vi "Is DaisyChain open.vi"(0 "System no.":i32=1 min=1 step=1, 5 "error in":errorcluster) -> (14 "PortID":i32, 15 "DC open?":bool, 19 "error out":errorcluster)   [LabVIEW 2020]
doc: "This VI checks if a DaisyChain connection is already open for the communication port defined for the given System no. It does also return the Port ID of the DaisyChain connection if any exists.\n\nE-709: Only supported if E-709 is used inside C-867K012/K013."
uses:
  ProgramData/PI/LabVIEW/Low Level/Communication.llb/Global DaisyChain.vi
  ProgramData/PI/LabVIEW/Low Level/Communication.llb/Global1.vi
panel:
  # "This vi checks if a DaisyChain connection is already open \nfor the selected interface."
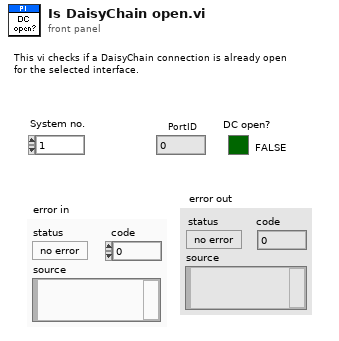
[diagram p1: front panel]
types:
  T1 = typedef "Available DLLs.ctl" = u16
  T2 = typedef "Available DLL interfaces.ctl" = u16
  T3 = cluster{"DLL for Device":T1, "DLL Interface":T2, "Parameter":string}[]
  T4 = typedef "Available interfaces.ctl" = u16
  T5 = cluster{"RS232 Portnumber":i32, "Timeout":i32, "RS232 Baud rate":u32, "Interface":T4, "GPIB Bus":i32, "GPIB Address":i32, "GPIB Mode":i32}[]
  T6 = cluster{"No. of devices":i32, "Port ID":i32, "Devices":string[], "Description":string}[]
  T7 = cluster{"RS232 Portnumber":i32, "Timeout":i32, "RS232 Baud rate":u32, "Interface":T4, "GPIB Bus":i32, "GPIB Address":i32, "GPIB Mode":i32}
  T8 = cluster{"DLL for Device":T1, "DLL Interface":T2, "Parameter":string}
  T9 = cluster{"No. of devices":i32, "Port ID":i32, "Devices":string[], "Description":string}
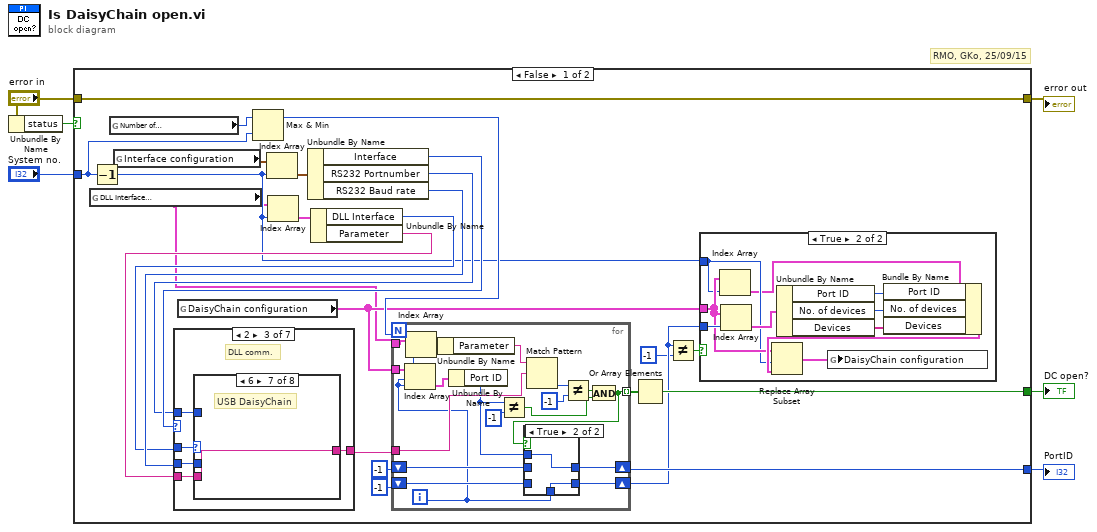
[diagram p0: block diagram]
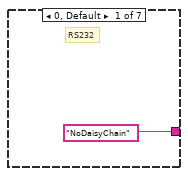
[diagram p3: hidden frame]
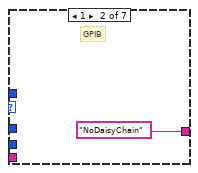
[diagram p4: hidden frame]
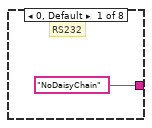
[diagram p5: hidden frame]
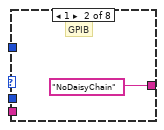
[diagram p6: hidden frame]
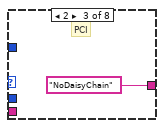
[diagram p7: hidden frame]
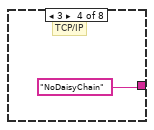
[diagram p8: hidden frame]
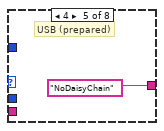
[diagram p9: hidden frame]
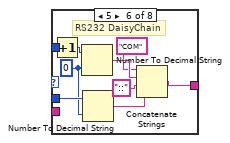
[diagram p10: hidden frame]
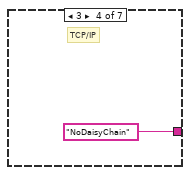
[diagram p12: hidden frame]
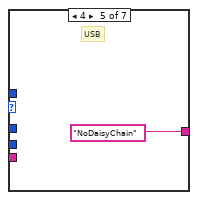
[diagram p13: hidden frame]
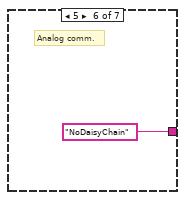
[diagram p14: hidden frame]
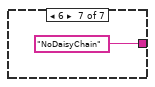
[diagram p15: hidden frame]
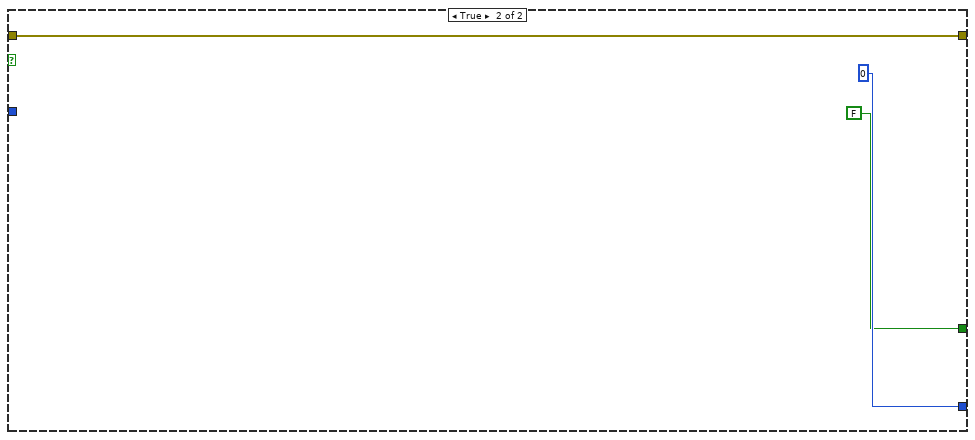
[diagram p17: hidden frame]
diagram:
  # "RMO, GKo, 25/09/15"
  n1 = Unbundle By Name("error in") -> ("status"=w5:bool)
  n2 = case shown="False" w5 {
    tunnel: [w22 w92] -> w4
    tunnel: "error in" -> [w22 w92]
    tunnel: [w26 0] -> w3
    tunnel: [w14 FALSE] -> w2
    tunnel: "System no." -> [w17 _]
    frame False {
      n3 = global read "Global1.vi" "DLL Interface\nConfiguration"() -> (w7:T3)
      n4 = Decrement(x=w17) -> (x-1=w8:i32)
      n5 = global read "Global1.vi" "Number of\nsystems"() -> (w18:i32)
      n6 = global read "Global1.vi" "Interface configuration"() -> (w30:T5)
      n7 = global read "Global DaisyChain.vi" "DaisyChain configuration"() -> (w9:T6)
      n8 = Max & Min(x=w18, y=w17) -> (max(x,y)=w16:i32)  [unwired: 1 out]
      n9 = Index Array(array=w30, index=w8) -> (element=w29:T7)
      n10 = Index Array(array=w7, index=w8) -> (element=w21:T8)
      n11 = Unbundle By Name(w29) -> ("Interface"=w25:T4, "RS232 Portnumber"=w24:i32, "RS232 Baud rate"=w23:u32)
      n12 = Unbundle By Name(w21) -> ("DLL Interface"=w20:T2, "Parameter"=w10:string)
      n13 = case shown="2" w25 {
        tunnel: ["NoDaisyChain" "NoDaisyChain" w47 "NoDaisyChain" "NoDaisyChain" "NoDaisyChain" "NoDaisyChain"] -> w19
        tunnel: w24 -> [_ _ w46 _ _ _ _]
        tunnel: w23 -> [_ _ w45 _ _ _ _]
        tunnel: w20 -> [_ _ w44 _ _ _ _]
        tunnel: w10 -> [_ _ w43 _ _ _ _]
        frame 0, Default {
          # "RS232"
        }
        frame 1 {
          # "GPIB"
        }
        frame 2 {
          # "DLL comm."
          n14 = case shown="6" w44 {
            tunnel: ["NoDaisyChain" "NoDaisyChain" "NoDaisyChain" "NoDaisyChain" "NoDaisyChain" w58 w62 w63] -> w47
            tunnel: w46 -> [_ _ _ _ _ w57 _ _]
            tunnel: w45 -> [_ _ _ _ _ w55 _ _]
            tunnel: w43 -> [_ _ _ _ _ _ w62 w63]
            frame 0, Default {
              # "RS232"
            }
            frame 1 {
              # "GPIB"
            }
            frame 2 {
              # "PCI"
            }
            frame 3 {
              # "TCP/IP"
            }
            frame 4 {
              # "USB (prepared)"
            }
            frame 5 {
              w54 = i16 0 ("width (-)")
              # "RS232 DaisyChain"
              n15 = Increment(x=w57) -> (x+1=w56:i32)
              n16 = Number To Decimal String(number=w56, width (-)=w54) -> (decimal integer string=w61:string)
              n17 = Number To Decimal String(number=w55, width (-)=w54) -> (decimal integer string=w59:string)
              n18 = Concatenate Strings("COM" ("string"), w61, "::" ("string"), w59) -> (w58:string)
            }
            frame 6 {
              # "USB DaisyChain"
            }
            frame 7 {
              # "TCPIP DaisyChain"
            }
          }
        }
        frame 3 {
          # "TCP/IP"
        }
        frame 4 {
          (unwired) refnum<visa-resource-name> refnum ("duplicate VISA resource name")
          (unwired) FALSE ("status")
          (unwired) 0 ("error code")
          (unwired) 0
          # "USB"
        }
        frame 5 {
          (unwired) refnum<visa-resource-name> refnum ("duplicate VISA resource name")
          (unwired) FALSE ("status")
          (unwired) 0 ("error code")
          (unwired) 0
          # "Analog comm."
        }
        frame 6 {
        }
      }
      n19 = for {
        N: w16 -> [_]
        tunnel: w9 -> [w73]
        tunnel: [w79] -> w28 mode=indexing
        shift-right: [w83] -> w26
        shift-left: -1 ("Port ID") -> [w82]
        tunnel: w19 -> [w81]
        shift-right: [w74] -> w13
        shift-left: -1 -> [w75]
        tunnel: w7 -> [w71]
        i -> [w72]
        n20 = Index Array(array=w73, index=w72) -> (element=w70:T9)
        n21 = Index Array(array=w71, index=w72) -> (element=w69:T8)
        n22 = Unbundle By Name(w69) -> ("Parameter"=w68:string)
        n23 = Unbundle By Name(w70) -> ("Port ID"=w77:i32)
        n24 = Not Equal?(x=w77, y=-1) -> (x != y?=w76:bool)
        n25 = Match Pattern(string=w68, regular expression=w81) -> (offset past match=w85:i32)  [unwired: 4 out]
        n26 = Not Equal?(x=w85, y=-1) -> (x != y?=w80:bool)
        n27 = And(x=w80, y=w76) -> (x .and. y?=w79:bool)
        n28 = case shown="True" w79 {
          tunnel: [w87 w89] -> w83
          tunnel: w77 -> [_ w89]
          tunnel: w82 -> [w87 _]
          tunnel: w75 -> [w86 _]
          tunnel: [w86 w88] -> w74
          tunnel: w72 -> [_ w88]
          frame False {
          }
          frame True {
          }
        }
      }
      n29 = Or Array Elements(Boolean array=w28) -> (logical OR=w14:bool)
      n30 = Not Equal?(x=w13, y=-1) -> (x != y?=w11:bool)
      n31 = case shown="True" w11 {
        tunnel: w9 -> [_ w33]
        tunnel: w13 -> [_ w40]
        tunnel: w8 -> [_ w32]
        frame False {
        }
        frame True {
          n32 = Index Array(array=w33, index=w32) -> (element=w31:T9)
          n33 = Index Array(array=w33, index=w40) -> (element=w37:T9)
          n34 = Unbundle By Name(w37) -> ("Port ID"=w36:i32, "No. of devices"=w35:i32, "Devices"=w34:string[])
          n35 = Bundle By Name(cluster=w31, "Port ID"=w36, "No. of devices"=w35, "Devices"=w34) -> (w38:T9)
          n36 = Replace Array Subset(array=w33, new element=w38, index=w32) -> (w39:T6)
          n37 = global write "Global DaisyChain.vi" "DaisyChain configuration"(w39) -> ()
        }
      }
    }
    frame True {
    }
  }
  "error out" <- w4
  "PortID" <- w3
  "DC open?" <- w2
